vi "overlayGUI.vi"(8 "error in (no error)":errorcluster) -> (0 "error out":errorcluster)   [LabVIEW 2010]
uses:
  common/classes/Image/Image/Image.lvclass
  <vilib>/vision/Image Controls.llb/IMAQ Image.ctl
  <vilib>/vision/NI_Vision_Development_Module.lvlib
panel:
  in  "quitButton":bool
  in  "clear text button":bool
  in  "label text":string
  in  "text button":bool
  in  "save button":bool
  in  "clearROIsButton":bool
  in  "load intrinsic button":bool
  in  "load reference button":bool
  out "intrinsic optical signal image":T1(plugin-control)
  out "reference image":T1(plugin-control)
  # "Intrinsic Optical Imaging: Overlay Tool"
  # "Procedure:\n1. Load a reference image (camera image with blood vessel pattern) and the intrinsic optical signal image.\n2. On the intrinsic optical signal image, draw and label regions. They will automatically be overlaid onto the reference image.\n3. Save the reference image with overlays."
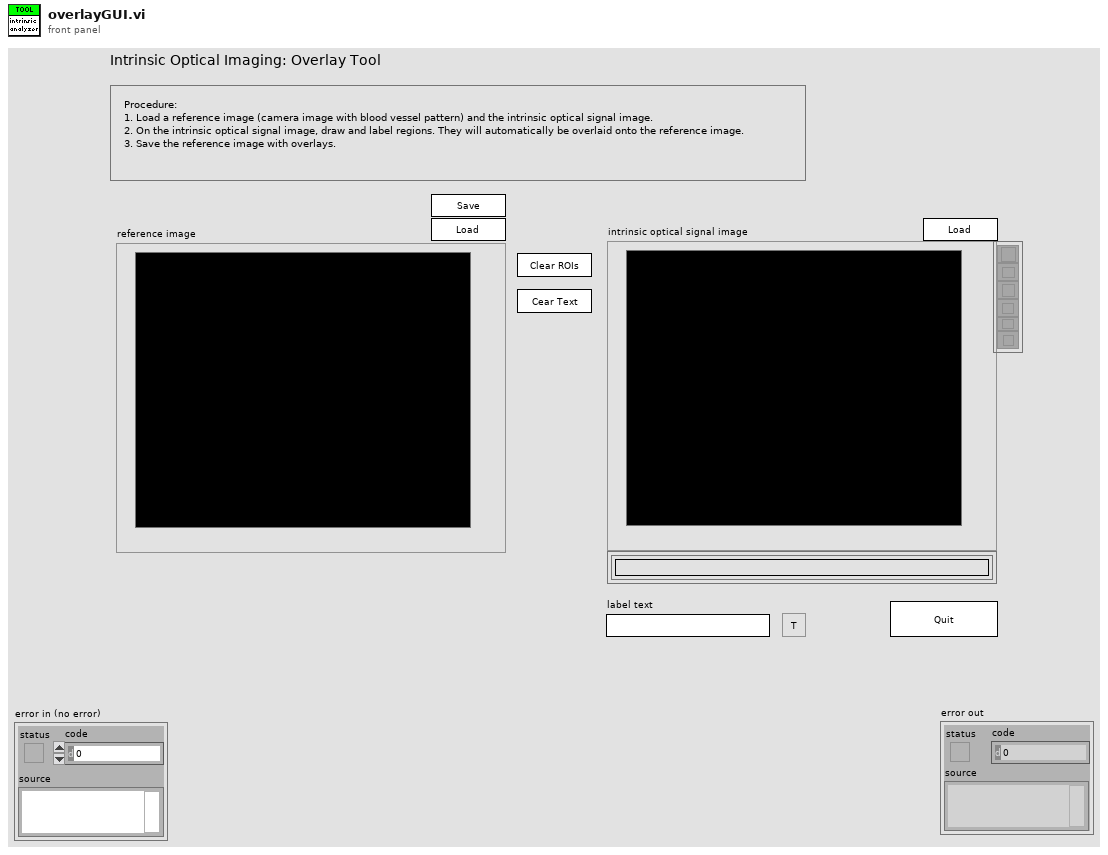
[diagram p1: front panel]
types:
  T1 = typedef "IMAQ Image.ctl" = refnum<image>
  T2 = cluster{"Desired Font (Application)":enum16{"User-specified Font", "Application Font", "System Font", "Dialog Font"}, "[User-specified Font]":cluster{"Font Name":string, "Size":i16, "Strikeout?":bool, "Italic?":bool, "Underline?":bool, "Outline?":bool, "Shadow?":bool, "Bold?":bool, "Rotation Angle":dbl}, "Horizontal Alignment":i16, "Vertical Alignment":i16}
  T3 = typedef "ROI Descriptor" = cluster{"Global Rectangle":i32[], "Contours":cluster{"ID":enum32{"External", "Internal"}, "Type":u32, "Coordinates":i32[]}[]}
  T4 = typedef "Image Type" = u32
  T5 = cluster{"Global Rectangle":i32[], "Contours":cluster{"Contour Type":u32, "ROI Type":u32, "Points":i32[]}[]}
  T6 = cluster{"Global Rectangle":i32[], "Contours":cluster{"Contour Type":u32, "ROI Type":u32, "Points":i32[]}[]}[]
  T7 = cluster{"Coordinates[0]":i32, "Coordinates[1]":i32}
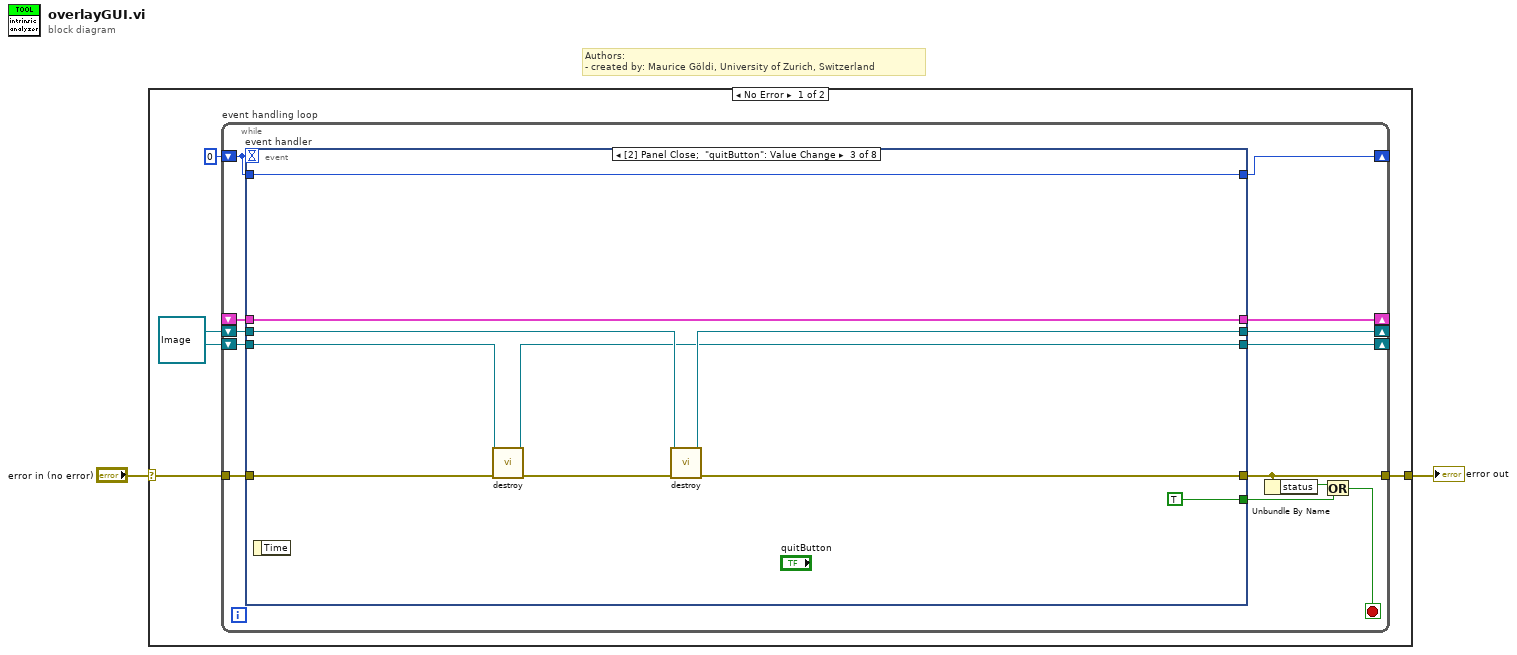
[diagram p0: block diagram]
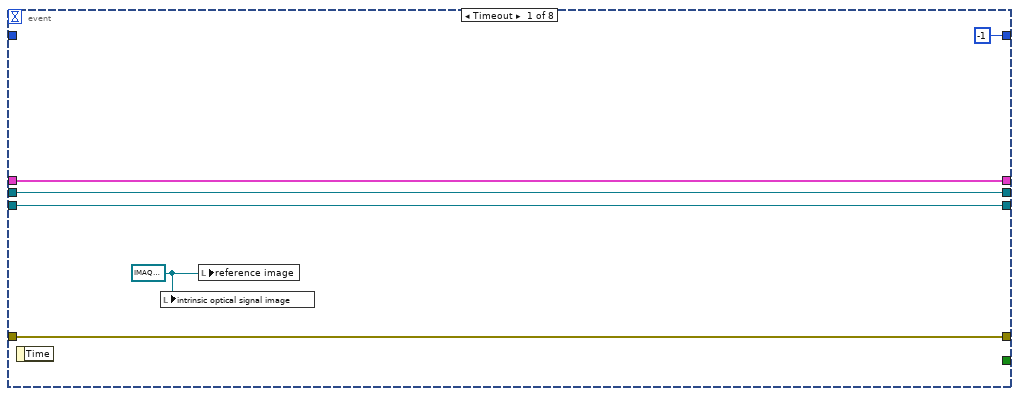
[diagram p2: hidden frame]
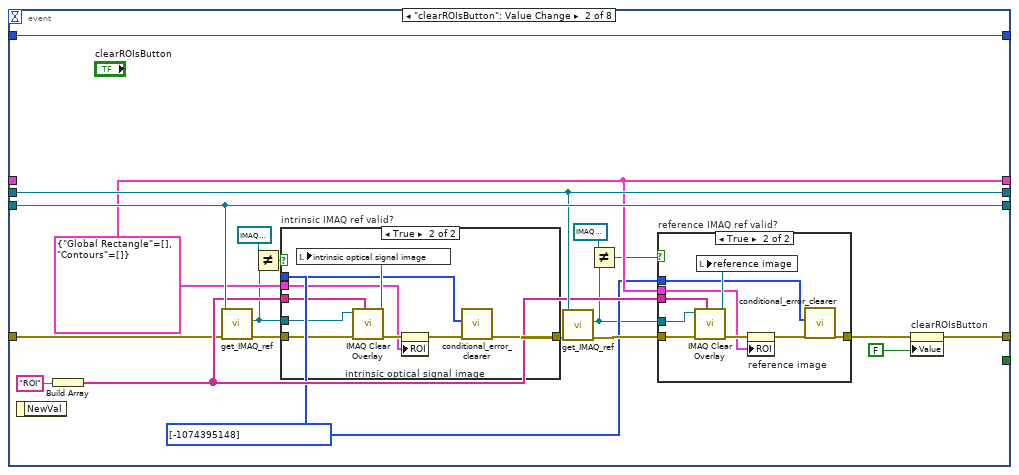
[diagram p3: hidden frame]
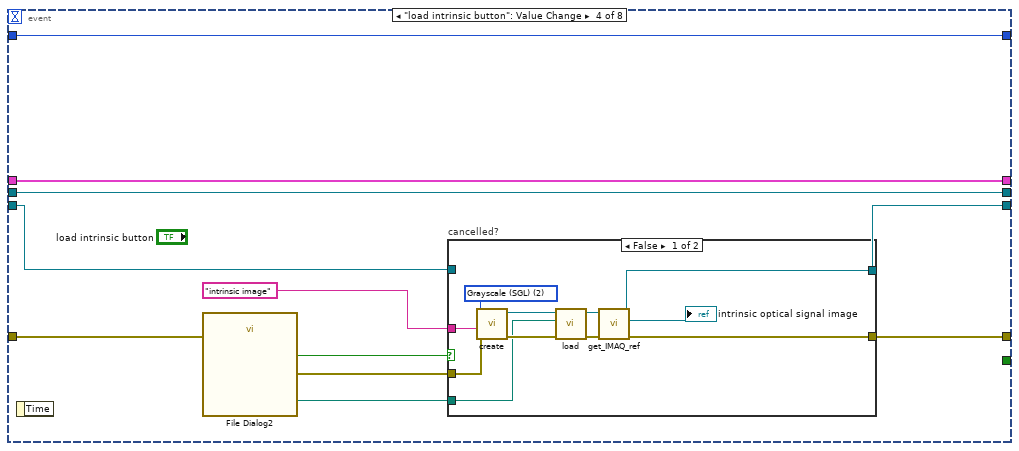
[diagram p6: hidden frame]
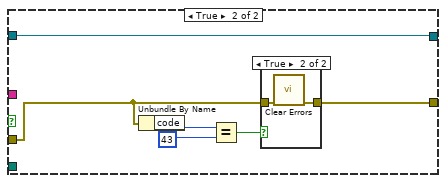
[diagram p7: hidden frame]
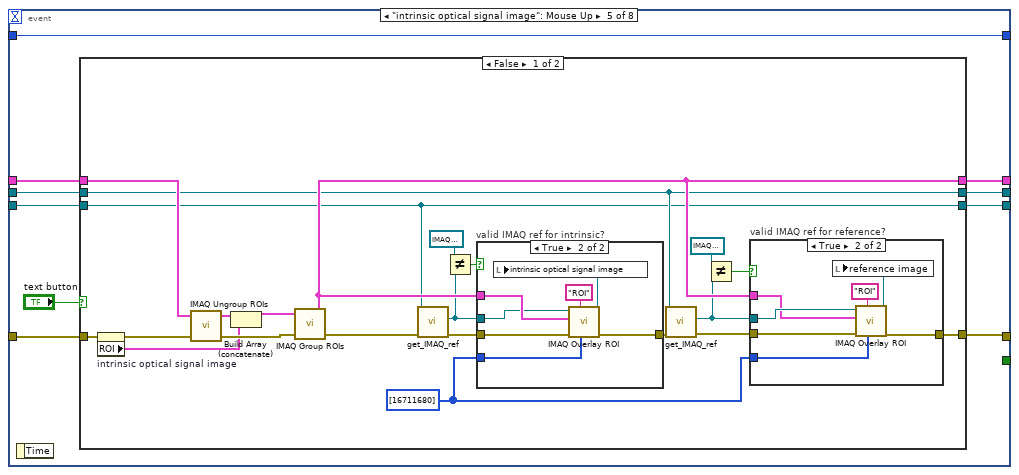
[diagram p9: hidden frame]
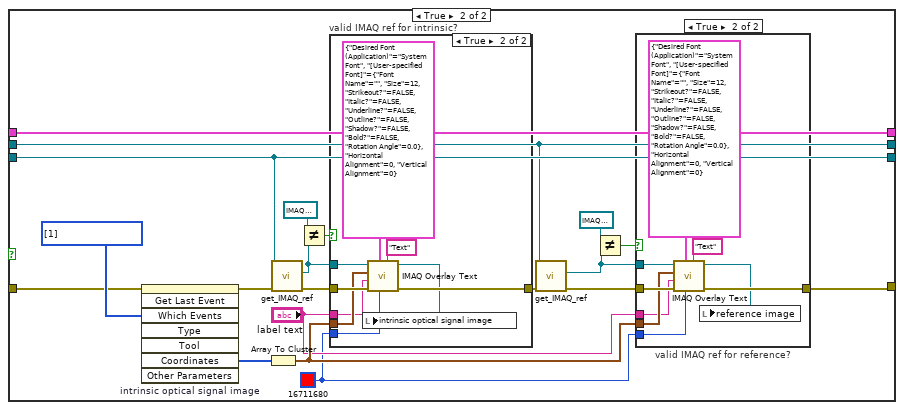
[diagram p12: hidden frame]
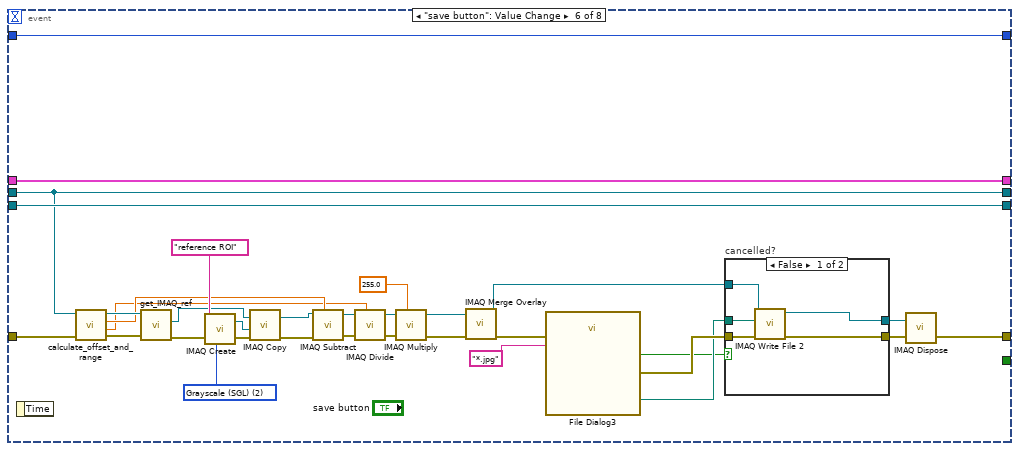
[diagram p15: hidden frame]
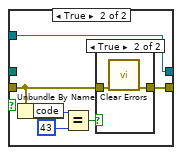
[diagram p16: hidden frame]
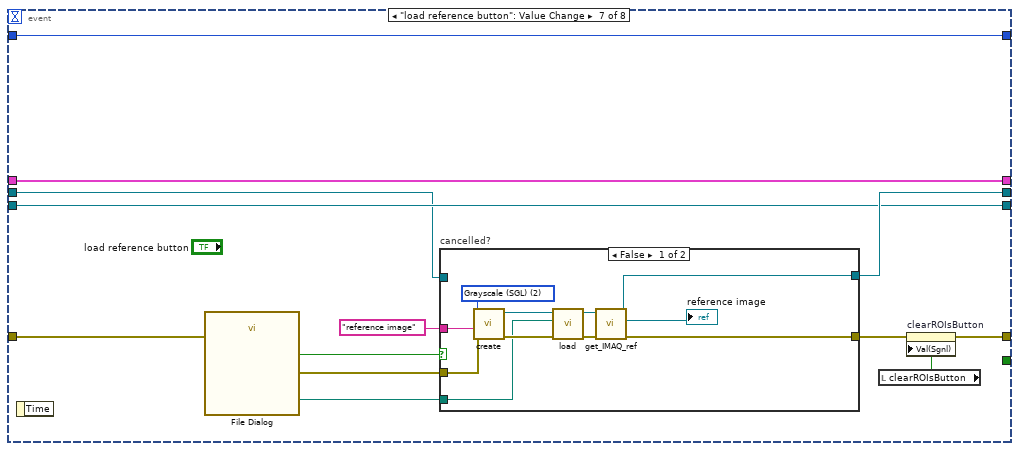
[diagram p18: hidden frame]
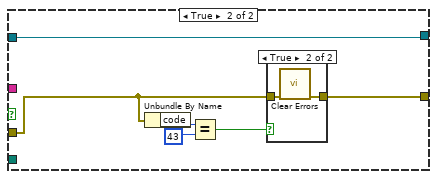
[diagram p19: hidden frame]
diagram:
  # "Authors: \n- created by: Maurice Göldi, University of Zurich, Switzerland"
  n1 = case shown="No Error" "error in (no error)" {
    selector: "error in (no error)" -> [w4 w304]
    tunnel: [w5 w304] -> w1
    frame No Error {
      w3 = refnum<class "Image.lvclass"> refnum ("Image.lvclass")
      n2 = while "event handling loop" {
        tunnel: [w11] -> w5
        shift-right: [w18] -> _
        shift-left: 0 -> [w19]
        shift-right: [w17] -> _
        shift-left: _ -> [w16]
        shift-right: [w15] -> _
        shift-left: w3 -> [w14]
        shift-right: [w12] -> _
        shift-left: w3 -> [w13]
        tunnel: w4 -> [w7]
        stop <- w9 stop-if-true
        n3 = event "event handler" shown="[2] Panel Close;  \"quitButton\": Value Change" {
          selector: _ -> [_ _ _ _ _ _ _ _]
          dyn-events: _ -> [_ _ _ _ _ _ _ _]
          timeout: w19 -> [_ _ _ _ _ _ _ _]
          tunnel: w19 -> [_ w45 w75 w86 w116 w227 w254 w291]
          tunnel: [_ _ TRUE _ _ _ _ _] -> w8
          tunnel: [w20 w35 w72 w84 w114 w217 w244 w283] -> w11
          tunnel: [-1 w45 w75 w86 w116 w227 w254 w291] -> w18
          tunnel: [w21 w37 w74 w81 w112 w225 w250 w290] -> w17
          tunnel: w16 -> [w21 _ w74 w81 w115 w225 w250 w290]
          tunnel: [w23 w41 w69 w79 w110 w212 w249 w282] -> w15
          tunnel: w14 -> [w23 w41 w70 w79 w108 w212 w247 w282]
          tunnel: w13 -> [w22 w44 w68 w78 w113 w226 w248 w281]
          tunnel: [w22 w44 w67 w80 w109 w226 w248 w281] -> w12
          tunnel: w7 -> [w20 w33 w73 w76 w107 w195 w242 w284]
          event Timeout {
            w24 = T1 refnum ("blood vessel image")
            n4 = event-data() -> ()  [unwired: 1 in, 1 out]
            n5 = local write "intrinsic optical signal image"(w24) -> ()
            n6 = local write "reference image"(w24) -> ()
          }
          event "clearROIsButton": Value Change {
            w32 = i32[] [-1074395148] ("array of clearable error codes")
            w37 = T3 {"Global Rectangle"=[], "Contours"=[]} ("ROI Descriptor out")
            n7 = event-data() -> ()  [unwired: 1 in, 1 out]
            n8 = Build Array("ROI" ("Group")) -> (w38:string[])
            n9 = call-dynamic "get_IMAQ_ref.vi"("error in (no error)"=w33, "Image.lvclass in"=w44) -> ("error out"=w43:errorcluster, "Image"=w27:T1)  [unwired: 5 in, 3 out]
            n10 = Not Equal?(x=T1 refnum, y=w27) -> (x != y?=w26:bool)
            n11 = case "intrinsic IMAQ ref valid?" shown="True" w26 {
              tunnel: w27 -> [_ w65]
              tunnel: w43 -> [w56 w64]
              tunnel: [w56 w58] -> w42
              tunnel: w38 -> [_ w62]
              tunnel: w37 -> [_ w60]
              tunnel: w32 -> [_ w57]
              frame False {
              }
              frame True {
                n12 = call "IMAQ Clear Overlay"("Groups"=w62, "error in (no error)"=w64, "Image"=w65) -> ("error out"=w61:errorcluster, "Image Out"=w63:T1)  [unwired: 7 in]
                n13 = local write "intrinsic optical signal image"(w63) -> ()
                n14 = property on="intrinsic optical signal image" class="ImageControl"(error in=w61, "ROI"=w60) -> (error out=w59:errorcluster)  [unwired: 1 in, 1 out]
                n15 = call "conditional_error_clearer.vi"("error in (no error)"=w59, "array of clearable error codes"=w57) -> ("error out"=w58:errorcluster)  [unwired: 9 in]
              }
            }
            n16 = call-dynamic "get_IMAQ_ref.vi"("error in (no error)"=w42, "Image.lvclass in"=w41) -> ("error out"=w40:errorcluster, "Image"=w30:T1)  [unwired: 5 in, 3 out]
            n17 = Not Equal?(x=T1 refnum, y=w30) -> (x != y?=w29:bool)
            n18 = case "reference IMAQ ref valid?" shown="True" w29 {
              tunnel: w40 -> [w46 w55]
              tunnel: [w46 w48] -> w34
              tunnel: w30 -> [_ w54]
              tunnel: w38 -> [_ w52]
              tunnel: w37 -> [_ w50]
              tunnel: w32 -> [_ w47]
              frame False {
              }
              frame True {
                n19 = call "IMAQ Clear Overlay"("Groups"=w52, "error in (no error)"=w55, "Image"=w54) -> ("error out"=w51:errorcluster, "Image Out"=w53:T1)  [unwired: 7 in]
                n20 = local write "reference image"(w53) -> ()
                n21 = property on="reference image" class="ImageControl"(error in=w51, "ROI"=w50) -> (error out=w49:errorcluster)  [unwired: 1 in, 1 out]
                n22 = call "conditional_error_clearer.vi"("error in (no error)"=w49, "array of clearable error codes"=w47) -> ("error out"=w48:errorcluster)  [unwired: 9 in]
              }
            }
            n23 = property on="clearROIsButton" class="Bool (strict)"(error in=w34, "Value"=FALSE) -> (error out=w35:errorcluster)  [unwired: 1 in, 1 out]
          }
          event Panel Close; "quitButton": Value Change {
            n24 = event-data() -> ()  [unwired: 1 in, 1 out]
            n25 = call-dynamic "destroy.vi"("error in (no error)"=w73, "Image in"=w68) -> ("error out"=w71:errorcluster, "Image out"=w67:refnum<class "Image.lvclass">)  [unwired: 8 in]
            n26 = call-dynamic "destroy.vi"("error in (no error)"=w71, "Image in"=w70) -> ("error out"=w72:errorcluster, "Image out"=w69:refnum<class "Image.lvclass">)  [unwired: 8 in]
          }
          event "load intrinsic button": Value Change {
            n27 = event-data() -> ()  [unwired: 1 in, 1 out]
            n28 = call "File Dialog2"("error in"=w76) -> ("selected path"=w83:path, "cancelled"=w77:bool, "error out"=w85:errorcluster)  [unwired: 11 in, 1 out]
            n29 = case "cancelled?" shown="False" w77 {
              tunnel: w85 -> [w92 w98]
              tunnel: [w91 w99] -> w84
              tunnel: w83 -> [w89 _]
              tunnel: "intrinsic image" ("name") -> [w88 _]
              tunnel: [w87 w103] -> w80
              tunnel: w78 -> [_ w103]
              frame False {
                w93 = T4 2 items=["Grayscale (U8)", "Grayscale (I16)", "Grayscale (SGL)", "Complex (CSG)", "RGB (U32)", "HSL (U32)", "RGB (U64)", "Grayscale (U16)"] ("Image Type")
                n30 = call "create.vi"("error in (no error)"=w92, "name"=w88, "Image Type"=w93) -> ("error out"=w97:errorcluster, "Image out"=w96:refnum<class "Image.lvclass">)  [unwired: 7 in]
                n31 = call-dynamic "load.vi"("error in (no error)"=w97, "Path"=w89, "Image in"=w96) -> ("error out"=w94:errorcluster, "Image out"=w95:refnum<class "Image.lvclass">)  [unwired: 5 in, 2 out]
                n32 = call-dynamic "get_IMAQ_ref.vi"("error in (no error)"=w94, "Image.lvclass in"=w95) -> ("error out"=w91:errorcluster, "Image"=→"intrinsic optical signal image":T1, "Image.lvclass out"=w87:refnum<class "Image.lvclass">)  [unwired: 5 in, 2 out]
              }
              frame True {
                n33 = Unbundle By Name(w98) -> ("code"=w100:i32)
                n34 = Equal?(x=w100, y=43) -> (x = y?=w102:bool)
                n35 = case shown="True" w102 {
                  tunnel: w98 -> [w104 w106]
                  tunnel: [w104 w105] -> w99
                  frame False {
                  }
                  frame True {
                    n36 = call <vilib>:"Clear Errors.vi"("error in (no error)"=w106) -> ("error out"=w105:errorcluster)  [unwired: 6 in]
                  }
                }
              }
            }
          }
          event "intrinsic optical signal image": Mouse Up {
            n37 = event-data() -> ()  [unwired: 1 in, 1 out]
            n38 = case shown="False" "text button" {
              tunnel: w115 -> [w135 w174]
              tunnel: [w131 w167] -> w114
              tunnel: w113 -> [w124 w173]
              tunnel: w108 -> [w125 w162]
              tunnel: [w126 w174] -> w112
              tunnel: [w125 w162] -> w110
              tunnel: [w124 w173] -> w109
              tunnel: w107 -> [w123 w168]
              frame False {
                w127 = u32[] [16711680] ("Colors (Green)")
                n39 = property on="intrinsic optical signal image" class="ImageControl"(error in=w123) -> (error out=w138:errorcluster, "ROI"=w133:T5)  [unwired: 1 in, 1 out]
                n40 = call "IMAQ Ungroup ROIs"("error in (no error)"=w138, "ROI Descriptor"=w135) -> ("error out"=w137:errorcluster, "ROI Descriptors out"=w134:T3[])  [unwired: 2 in]
                n41 = Build Array (concatenate)(w134, w133) -> (w136:T6)
                n42 = call "IMAQ Group ROIs"("error in (no error)"=w137, "ROI Descriptors"=w136) -> ("error out"=w132:errorcluster, "ROI Descriptor out"=w126:T3)  [unwired: 2 in]
                n43 = call-dynamic "get_IMAQ_ref.vi"("error in (no error)"=w132, "Image.lvclass in"=w124) -> ("error out"=w130:errorcluster, "Image"=w121:T1)  [unwired: 5 in, 3 out]
                n44 = Not Equal?(x=T1 refnum, y=w121) -> (x != y?=w120:bool)
                n45 = case "valid IMAQ ref for intrinsic?" shown="True" w120 {
                  tunnel: w126 -> [_ w154]
                  tunnel: w130 -> [w147 w153]
                  tunnel: w121 -> [_ w152]
                  tunnel: [w147 w151] -> w128
                  tunnel: w127 -> [_ w149]
                  frame False {
                  }
                  frame True {
                    n46 = call "IMAQ Overlay ROI"("Colors (Green)"=w149, "Group"="ROI", "error in (no error)"=w153, "ROI Descriptor"=w154, "Image"=w152) -> ("error out"=w151:errorcluster, "Image Out"=w150:T1)  [unwired: 5 in]
                    n47 = local write "intrinsic optical signal image"(w150) -> ()
                  }
                }
                n48 = call-dynamic "get_IMAQ_ref.vi"("error in (no error)"=w128, "Image.lvclass in"=w125) -> ("error out"=w129:errorcluster, "Image"=w118:T1)  [unwired: 5 in, 3 out]
                n49 = Not Equal?(x=T1 refnum, y=w118) -> (x != y?=w117:bool)
                n50 = case "valid IMAQ ref for reference?" shown="True" w117 {
                  tunnel: [w139 w146] -> w131
                  tunnel: w129 -> [w139 w145]
                  tunnel: w118 -> [_ w144]
                  tunnel: w127 -> [_ w142]
                  tunnel: w126 -> [_ w141]
                  frame False {
                  }
                  frame True {
                    n51 = call "IMAQ Overlay ROI"("Colors (Green)"=w142, "Group"="ROI", "error in (no error)"=w145, "ROI Descriptor"=w141, "Image"=w144) -> ("error out"=w146:errorcluster, "Image Out"=w143:T1)  [unwired: 5 in]
                    n52 = local write "reference image"(w143) -> ()
                  }
                }
              }
              frame True {
                w161 = u32 16711680 ("Text Color (black)")
                w169 = i32[] [1] items=["No  event", "Click event", "Draw event", "Move event", "Size event", "Scroll event", "Activate event", "Close event", "Double click event"] ("Events list (all)")
                n53 = invoke on="intrinsic optical signal image" class="ImageControl" method="Get Last Event"(error in=w168, "Which Events"=w169) -> (error out=w172:errorcluster, "Coordinates"=w170:i32[])  [unwired: 6 in, 6 out]
                n54 = Array To Cluster(array=w170) -> (cluster=w166:T7)
                n55 = call-dynamic "get_IMAQ_ref.vi"("error in (no error)"=w172, "Image.lvclass in"=w173) -> ("error out"=w171:errorcluster, "Image"=w156:T1)  [unwired: 5 in, 3 out]
                n56 = Not Equal?(x=T1 refnum, y=w156) -> (x != y?=w155:bool)
                n57 = case "valid IMAQ ref for intrinsic?" shown="True" w155 {
                  tunnel: [w185 w194] -> w163
                  tunnel: w171 -> [w185 w192]
                  tunnel: w156 -> [_ w191]
                  tunnel: w166 -> [_ w190]
                  tunnel: "label text" -> [_ w189]
                  tunnel: w161 -> [_ w186]
                  frame False {
                  }
                  frame True {
                    n58 = call "IMAQ Overlay Text"("Group"="Text", "Text Color (black)"=w186, "Font, Size & Style"=T2 {"Desired Font (Application)"=enum."System Font", "[User-specified Font]"={"Font Name"="", "Size"=12, "Strikeout?"=FALSE, "Italic?"=FALSE, "Underline?"=FALSE, "Outline?"=FALSE, "Shadow?"=FALSE, "Bold?"=FALSE, "Rotation Angle"=0.0}, "Horizontal Alignment"=0, "Vertical Alignment"=0}, "error in (no error)"=w192, "String"=w189, "Origin"=w190, "Image"=w191) -> ("error out"=w194:errorcluster, "Image Out"=w187:T1)  [unwired: 3 in]
                    n59 = local write "intrinsic optical signal image"(w187) -> ()
                  }
                }
                n60 = call-dynamic "get_IMAQ_ref.vi"("error in (no error)"=w163, "Image.lvclass in"=w162) -> ("error out"=w164:errorcluster, "Image"=w159:T1)  [unwired: 5 in, 3 out]
                n61 = Not Equal?(x=T1 refnum, y=w159) -> (x != y?=w160:bool)
                n62 = case "valid IMAQ ref for reference?" shown="True" w160 {
                  tunnel: [w175 w184] -> w167
                  tunnel: w164 -> [w175 w182]
                  tunnel: w159 -> [_ w181]
                  tunnel: w166 -> [_ w180]
                  tunnel: "label text" -> [_ w179]
                  tunnel: w161 -> [_ w176]
                  frame False {
                  }
                  frame True {
                    n63 = call "IMAQ Overlay Text"("Group"="Text", "Text Color (black)"=w176, "Font, Size & Style"=T2 {"Desired Font (Application)"=enum."System Font", "[User-specified Font]"={"Font Name"="", "Size"=12, "Strikeout?"=FALSE, "Italic?"=FALSE, "Underline?"=FALSE, "Outline?"=FALSE, "Shadow?"=FALSE, "Bold?"=FALSE, "Rotation Angle"=0.0}, "Horizontal Alignment"=0, "Vertical Alignment"=0}, "error in (no error)"=w182, "String"=w179, "Origin"=w180, "Image"=w181) -> ("error out"=w184:errorcluster, "Image Out"=w177:T1)  [unwired: 3 in]
                    n64 = local write "reference image"(w177) -> ()
                  }
                }
              }
            }
          }
          event "save button": Value Change {
            w213 = T4 2 items=["Grayscale (U8)", "Grayscale (I16)", "Grayscale (SGL)", "Complex (CSG)", "RGB (U32)", "HSL (U32)", "RGB (U64)", "Grayscale (U16)"] ("Image Type")
            n65 = event-data() -> ()  [unwired: 1 in, 1 out]
            n66 = call-dynamic "calculate_offset_and_range.vi"("error in (no error)"=w195, "Image in"=w212) -> ("error out"=w209:errorcluster, "range"=w198:dbl, "offset / minimum"=w199:dbl, "Image out"=w208:refnum<class "Image.lvclass">)  [unwired: 5 in, 1 out]
            n67 = call-dynamic "get_IMAQ_ref.vi"("error in (no error)"=w209, "Image.lvclass in"=w208) -> ("error out"=w214:errorcluster, "Image"=w201:T1)  [unwired: 5 in, 3 out]
            n68 = call "IMAQ Create"("Image Name"="reference ROI" ("description"), "Image Type"=w213, "error in (no error)"=w214) -> ("New Image"=w202:T1, "error out"=w205:errorcluster)  [unwired: 2 in]
            n69 = call "IMAQ Copy"("error in (no error)"=w205, "Image Dst"=w202, "Image Src"=w201) -> ("error out"=w204:errorcluster, "Image Dst Out"=w200:T1)  [unwired: 3 in]
            n70 = call "IMAQ Subtract"("Image Src A"=w200, "Constant"=w199, "error in (no error)"=w204) -> ("Image Dst Out"=w206:T1, "error out"=w207:errorcluster)  [unwired: 4 in]
            n71 = call "IMAQ Divide"("Image Src A"=w206, "Constant"=w198, "error in (no error)"=w207) -> ("Image Dst Out"=w211:T1, "error out"=w210:errorcluster)  [unwired: 4 in]
            n72 = call "IMAQ Multiply"("Image Src A"=w211, "Constant"=sgl 255.0, "error in (no error)"=w210) -> ("Image Dst Out"=w196:T1, "error out"=w203:errorcluster)  [unwired: 4 in]
            n73 = call "IMAQ Merge Overlay"("error in (no error)"=w203, "Image Src"=w196) -> ("error out"=w222:errorcluster, "Image Dst Out"=w223:T1)  [unwired: 8 in]
            n74 = call "File Dialog3"("error in"=w222, "pattern (all files)"="*.jpg" ("pattern label")) -> ("selected path"=w220:path, "cancelled"=w219:bool, "error out"=w221:errorcluster)  [unwired: 10 in, 1 out]
            n75 = case "cancelled?" shown="False" w219 {
              tunnel: [w229 w234] -> w216
              tunnel: w223 -> [w232 w238]
              tunnel: w221 -> [w231 w235]
              tunnel: w220 -> [w230 _]
              tunnel: [w228 w238] -> w218
              frame False {
                n76 = call-poly "IMAQ Write File 2"("error in (no error)"=w231, "File Path"=w230, "Image"=w232) -> ("error out"=w229:errorcluster, "Image Out (duplicate)"=w228:T1)  [unwired: 7 in]
              }
              frame True {
                n77 = Unbundle By Name(w235) -> ("code"=w237:i32)
                n78 = Equal?(x=w237, y=43) -> (x = y?=w233:bool)
                n79 = case shown="True" w233 {
                  tunnel: w235 -> [w239 w241]
                  tunnel: [w239 w240] -> w234
                  frame False {
                  }
                  frame True {
                    n80 = call <vilib>:"Clear Errors.vi"("error in (no error)"=w241) -> ("error out"=w240:errorcluster)  [unwired: 6 in]
                  }
                }
              }
            }
            n81 = call "IMAQ Dispose"("Image"=w218, "error in (no error)"=w216) -> ("error out"=w217:errorcluster)  [unwired: 4 in]
          }
          event "load reference button": Value Change {
            n82 = event-data() -> ()  [unwired: 1 in, 1 out]
            n83 = call "File Dialog"("error in"=w242) -> ("selected path"=w252:path, "cancelled"=w246:bool, "error out"=w251:errorcluster)  [unwired: 11 in, 1 out]
            n84 = case "cancelled?" shown="False" w246 {
              tunnel: "reference image" ("Image Name") -> [w264 _]
              tunnel: w252 -> [w263 _]
              tunnel: w251 -> [w261 w266]
              tunnel: [w258 w270] -> w243
              tunnel: [w255 w271] -> w249
              tunnel: w247 -> [_ w271]
              frame False {
                w256 = T4 2 items=["Grayscale (U8)", "Grayscale (I16)", "Grayscale (SGL)", "Complex (CSG)", "RGB (U32)", "HSL (U32)", "RGB (U64)", "Grayscale (U16)"] ("Image Type")
                n85 = call "create.vi"("error in (no error)"=w261, "name"=w264, "Image Type"=w256) -> ("error out"=w265:errorcluster, "Image out"=w262:refnum<class "Image.lvclass">)  [unwired: 7 in]
                n86 = call-dynamic "load.vi"("error in (no error)"=w265, "Path"=w263, "Image in"=w262) -> ("error out"=w259:errorcluster, "Image out"=w260:refnum<class "Image.lvclass">)  [unwired: 5 in, 2 out]
                n87 = call-dynamic "get_IMAQ_ref.vi"("error in (no error)"=w259, "Image.lvclass in"=w260) -> ("error out"=w258:errorcluster, "Image"=→"reference image":T1, "Image.lvclass out"=w255:refnum<class "Image.lvclass">)  [unwired: 5 in, 2 out]
              }
              frame True {
                n88 = Unbundle By Name(w266) -> ("code"=w267:i32)
                n89 = Equal?(x=w267, y=43) -> (x = y?=w269:bool)
                n90 = case shown="True" w269 {
                  tunnel: w266 -> [w272 w274]
                  tunnel: [w272 w273] -> w270
                  frame False {
                  }
                  frame True {
                    n91 = call <vilib>:"Clear Errors.vi"("error in (no error)"=w274) -> ("error out"=w273:errorcluster)  [unwired: 6 in]
                  }
                }
              }
            }
            n92 = local read "clearROIsButton"() -> (w245:bool)
            n93 = property on="clearROIsButton" class="Bool (strict)"(error in=w243, "Val(Sgnl)"=w245) -> (error out=w244:errorcluster)  [unwired: 1 in, 1 out]
          }
          event "clear text button": Value Change {
            n94 = event-data() -> ()  [unwired: 1 in, 3 out]
            n95 = Build Array("Text" ("Group")) -> (w285:string[])
            n96 = call-dynamic "get_IMAQ_ref.vi"("error in (no error)"=w284, "Image.lvclass in"=w281) -> ("error out"=w289:errorcluster, "Image"=w276:T1)  [unwired: 5 in, 3 out]
            n97 = Not Equal?(x=T1 refnum, y=w276) -> (x != y?=w275:bool)
            n98 = case "valid IMAQ ref for intrinsic?" shown="True" w275 {
              tunnel: w276 -> [_ w303]
              tunnel: w289 -> [w298 w302]
              tunnel: [w298 w301] -> w288
              tunnel: w285 -> [_ w300]
              frame False {
              }
              frame True {
                n99 = call "IMAQ Clear Overlay"("Groups"=w300, "error in (no error)"=w302, "Image"=w303) -> ("error out"=w301:errorcluster, "Image Out"=w299:T1)  [unwired: 7 in]
                n100 = local write "intrinsic optical signal image"(w299) -> ()
              }
            }
            n101 = call-dynamic "get_IMAQ_ref.vi"("error in (no error)"=w288, "Image.lvclass in"=w282) -> ("error out"=w287:errorcluster, "Image"=w279:T1)  [unwired: 5 in, 3 out]
            n102 = Not Equal?(x=T1 refnum, y=w279) -> (x != y?=w278:bool)
            n103 = case "valid IMAQ ref for reference?" shown="True" w278 {
              tunnel: w287 -> [w292 w297]
              tunnel: [w292 w296] -> w283
              tunnel: w279 -> [_ w295]
              tunnel: w285 -> [_ w294]
              frame False {
              }
              frame True {
                n104 = call "IMAQ Clear Overlay"("Groups"=w294, "error in (no error)"=w297, "Image"=w295) -> ("error out"=w296:errorcluster, "Image Out"=w293:T1)  [unwired: 7 in]
                n105 = local write "reference image"(w293) -> ()
              }
            }
          }
        }
        n106 = Unbundle By Name(w11) -> ("status"=w10:bool)
        n107 = Or(x=w10, y=w8) -> (x .or. y?=w9:bool)
      }
    }
    frame Error {
    }
  }
  "error out" <- w1
